vi "Set Strings from Ref.vi"(8 "error in (no error)":errorcluster, 9 "Language Index (0)":i32, 10 "GObj Refnum":refnum<vi>, 11 "GObject in":refnum<class "GObject.lvclass">) -> (0 "error out":errorcluster, 3 "GObject out":refnum<class "GObject.lvclass">)   [LabVIEW 2013, in "SET Project Data.lvlib" / "GObject.lvclass"]
uses:
  GObject.lvclass
  GObject.lvclass/GObject.ctl
  <vilib>/ErrorRing/Error Ring.xnode
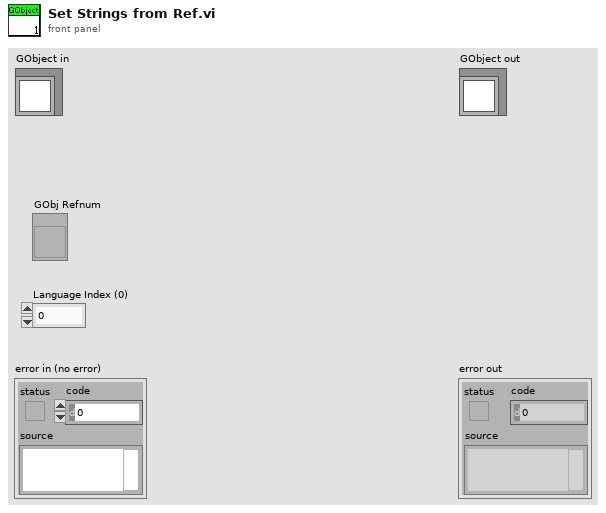
[diagram p1: front panel]
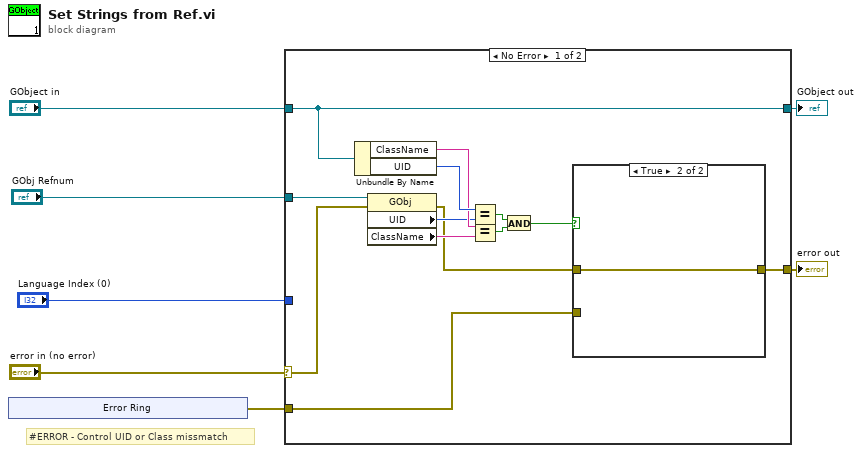
[diagram p0: block diagram]
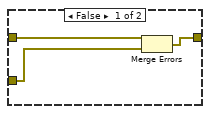
[diagram p2: hidden frame]
diagram:
  # "#ERROR - Control UID or Class missmatch"
  n1 = xnode "Error Ring"() -> ("error out"=w1:errorcluster)
  n2 = case shown="No Error" "error in (no error)" {
    selector: "error in (no error)" -> [w12 w26]
    tunnel: [w9 w26] -> w6
    tunnel: [w14 w25] -> w5
    tunnel: "GObject in" -> [w14 w25]
    tunnel: "Language Index (0)" -> [_ _]
    tunnel: "GObj Refnum" -> [w13 _]
    tunnel: w1 -> [w8 _]
    frame No Error {
      n3 = Unbundle By Name(w14) -> ("ClassName"=w17:string, "UID"=w18:i32)
      n4 = property class="GObj"(reference=w13, error in=w12) -> (error out=w10:errorcluster, "UID"=w15:i32, "ClassName"=w16:string)  [unwired: 1 out]
      n5 = Equal?(x=w18, y=w15) -> (x = y?=w20:bool)
      n6 = Equal?(x=w17, y=w16) -> (x = y?=w19:bool)
      n7 = And(x=w20, y=w19) -> (x .and. y?=w11:bool)
      n8 = case shown="True" w11 {
        tunnel: w10 -> [w23 w24]
        tunnel: [w22 w24] -> w9
        tunnel: w8 -> [w21 _]
        frame False {
          n9 = Merge Errors(w23, w21) -> (w22:errorcluster)
        }
        frame True {
        }
      }
    }
    frame Error {
    }
  }
  "error out" <- w6
  "GObject out" <- w5
